vi "NIIE_PictureControl_MouseUp.vi"(7 "Finalize Movement":bool, 8 "Error":errorcluster, 10 "Coords":T5, 11 "Data":T1={"Class"={"Ants"=refnum, "Layer"=refnum, "Templates"=refnum, "Icon"=refnum, "Glyph"=refnum, "Settings"=refnum, "Tools"=refnum}, "Ref"={"Add Layer"=refnum, "Remove Layer"=refnum, "Line Text"=[], "Body Text Spec"=refnum, "DNL_Font"=refnum, "glyph path str"=refnum, "templates path str"=refnum, "Arrow Up"=refnum, "Arrow Down"=refnum, "IE VI Ref"=refnum, "Glyphs tree"=refnum, "Templates tree"=refnum, "Layer Icon Text"=refnum, "Layer Template"=refnum, "Clipboard"=refnum, "BW icon in"=refnum, "Color icon in"=refnum, "Layer Clust"=refnum, "Body Text"=refnum, "DNL_Framework Templates"=refnum, "Search Templates"=refnum, "TextMarker"=refnum, "Tab Control"=refnum, "Search Glyphs"=refnum, "Line Color"=refnum, "DNL_Glyphs []"=refnum, "Fill Color"=refnum, "Tools"=refnum, "Glyphs tree"=refnum, "Icon"=refnum, "Preview"=refnum, "Ants"=refnum, "Terminals"=refnum, "menu reference"=refnum, "LayerNames"=[], "GlyphLoadAnimation"=refnum, "TemplateLoadAnimation"=refnum, "refreshGlyphs"=refnum, "refreshTemplates"=refnum}, "Support"={"AntsRect"={"left"=0, "top"=0, "right"=0, "bottom"=0}, "Mouse Move Coords"={"Horizontal"=0, "Vertical"=0}, "Mouse Down Coords"={"Horizontal"=0, "Vertical"=0}, "Temp Coord"={"Horizontal"=0, "Vertical"=0}, "Action"=enum."Default", "Edge Color"=4914962, "Fill Color"=16860, "Mouse Down?"=FALSE, "Draft Mode?"=FALSE, "Temp Icon"=bytes[3102], "CTRL Pressed"=FALSE, "Move Selection?"=FALSE, "AntsRect Orig"={"left"=0, "top"=0, "right"=0, "bottom"=0}, "Text"="", "TM Set?"=FALSE, "Mouse inside icon?"=FALSE, "Tool (old value)"=0, "Pencil Move Color"=0, "Swap Colors?"=FALSE, "Shift pressed?"=FALSE}}) -> (0 "Error Out":errorcluster, 3 "Data Out":T1={"Class"={"Ants"=refnum, "Layer"=refnum, "Templates"=refnum, "Icon"=refnum, "Glyph"=refnum, "Settings"=refnum, "Tools"=refnum}, "Ref"={"Add Layer"=refnum, "Remove Layer"=refnum, "Line Text"=[], "Body Text Spec"=refnum, "DNL_Font"=refnum, "glyph path str"=refnum, "templates path str"=refnum, "Arrow Up"=refnum, "Arrow Down"=refnum, "IE VI Ref"=refnum, "Glyphs tree"=refnum, "Templates tree"=refnum, "Layer Icon Text"=refnum, "Layer Template"=refnum, "Clipboard"=refnum, "BW icon in"=refnum, "Color icon in"=refnum, "Layer Clust"=refnum, "Body Text"=refnum, "DNL_Framework Templates"=refnum, "Search Templates"=refnum, "TextMarker"=refnum, "Tab Control"=refnum, "Search Glyphs"=refnum, "Line Color"=refnum, "DNL_Glyphs []"=refnum, "Fill Color"=refnum, "Tools"=refnum, "Glyphs tree"=refnum, "Icon"=refnum, "Preview"=refnum, "Ants"=refnum, "Terminals"=refnum, "menu reference"=refnum, "LayerNames"=[], "GlyphLoadAnimation"=refnum, "TemplateLoadAnimation"=refnum, "refreshGlyphs"=refnum, "refreshTemplates"=refnum}, "Support"={"AntsRect"={"left"=0, "top"=0, "right"=0, "bottom"=0}, "Mouse Move Coords"={"Horizontal"=0, "Vertical"=0}, "Mouse Down Coords"={"Horizontal"=0, "Vertical"=0}, "Temp Coord"={"Horizontal"=0, "Vertical"=0}, "Action"=enum."Default", "Edge Color"=4914962, "Fill Color"=16860, "Mouse Down?"=FALSE, "Draft Mode?"=FALSE, "Temp Icon"=bytes[3102], "CTRL Pressed"=FALSE, "Move Selection?"=FALSE, "AntsRect Orig"={"left"=0, "top"=0, "right"=0, "bottom"=0}, "Text"="", "TM Set?"=FALSE, "Mouse inside icon?"=FALSE, "Tool (old value)"=0, "Pencil Move Color"=0, "Swap Colors?"=FALSE, "Shift pressed?"=FALSE}})   [LabVIEW 2021]
uses:
  <vilib>/Utility/miscctls.llb/LVPoint32TypeDef.ctl
  Controls/IE Data.ctl
  Class/Ants/Ants.lvclass
  Class/FakedArray/FakedArray.lvclass
  Class/Icon Library/Glyph.lvclass
  Class/Settings/Settings.lvclass
  Class/Tools/Tools Paint.lvclass
  vi.lib/LabVIEW Icon API/lv_icon/Classes/Icon/Icon.lvclass
  Controls/IE Classes.ctl
  Controls/References Cluster.ctl
  Controls/SupportClass.ctl
  Controls/ENUM_SupportClass_Action.ctl
  vi.lib/LabVIEW Icon API/lv_icon/Controls/IEColor.ctl
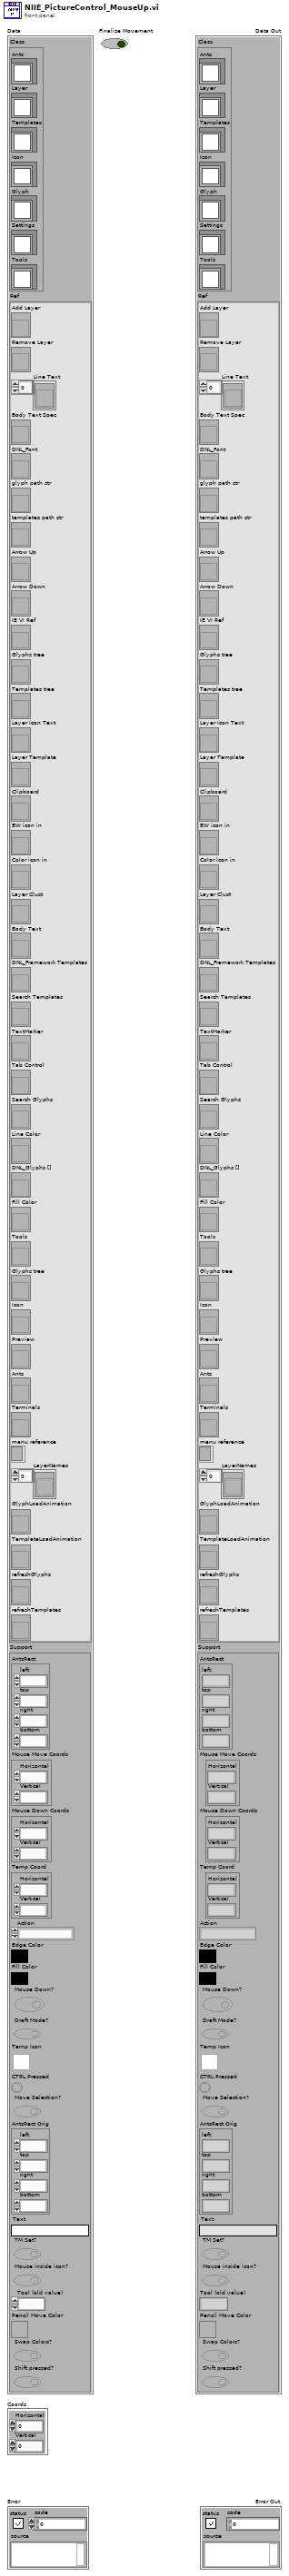
[diagram p1: front panel]
types:
  T1 = typedef "IE Data.ctl" = cluster{"Class":T2, "Ref":T3, "Support":T4}
  T2 = typedef "IE Classes.ctl" = cluster{"Ants":refnum<class "Ants.lvclass">, "Layer":refnum<class "FakedArray.lvclass">, "Templates":refnum<class "FakedArray.lvclass">, "Icon":refnum<class "Icon.lvclass">, "Glyph":refnum<class "Glyph.lvclass">, "Settings":refnum<class "Settings.lvclass">, "Tools":refnum<class "Tools Paint.lvclass">}
  T3 = typedef "References Cluster.ctl" = cluster{"Add Layer":refnum<vi>, "Remove Layer":refnum<vi>, "Line Text":refnum<vi>[], "Body Text Spec":refnum<vi>, "DNL_Font":refnum<vi>, "glyph path str":refnum<vi>, "templates path str":refnum<vi>, "Arrow Up":refnum<vi>, "Arrow Down":refnum<vi>, "IE VI Ref":refnum<vi>, "Glyphs tree":refnum<vi>, "Templates tree":refnum<vi>, "Layer Icon Text":refnum<vi>, "Layer Template":refnum<vi>, "Clipboard":refnum<vi>, "BW icon in":refnum<vi>, "Color icon in":refnum<vi>, "Layer Clust":refnum<vi>, "Body Text":refnum<vi>, "DNL_Framework Templates":refnum<vi>, "Search Templates":refnum<vi>, "TextMarker":refnum<vi>, "Tab Control":refnum<vi>, "Search Glyphs":refnum<vi>, "Line Color":refnum<vi>, "DNL_Glyphs []":refnum<vi>, "Fill Color":refnum<vi>, "Tools":refnum<vi>, "Glyphs tree":refnum<vi>, "Icon":refnum<vi>, "Preview":refnum<vi>, "Ants":refnum<vi>, "Terminals":refnum<vi>, "menu reference":refnum<k9>, "LayerNames":refnum<vi>[], "GlyphLoadAnimation":refnum<vi>, "TemplateLoadAnimation":refnum<vi>, "refreshGlyphs":refnum<vi>, "refreshTemplates":refnum<vi>}
  T4 = typedef "SupportClass.ctl" = cluster{"AntsRect":cluster{"left":i16, "top":i16, "right":i16, "bottom":i16}, "Mouse Move Coords":T5, "Mouse Down Coords":T5, "Temp Coord":T5, "Action":T6, "Edge Color":T7, "Fill Color":T7, "Mouse Down?":bool, "Draft Mode?":bool, "Temp Icon":picture, "CTRL Pressed":bool, "Move Selection?":bool, "AntsRect Orig":cluster{"left":i16, "top":i16, "right":i16, "bottom":i16}, "Text":string, "TM Set?":bool, "Mouse inside icon?":bool, "Tool (old value)":u32, "Pencil Move Color":u32, "Swap Colors?":bool, "Shift pressed?":bool}
  T5 = typedef "LVPoint32TypeDef.ctl" = cluster{"Horizontal":i32, "Vertical":i32}
  T6 = typedef "ENUM_SupportClass_Action.ctl" = enum16{"Default", "Move Selection", "Glyph Library", "Tool"}
  T7 = typedef "IEColor.ctl" = u32
  T8 = cluster{"left":i16, "top":i16, "right":i16, "bottom":i16}
  T9 = cluster{"Horizontal":i32, "Vertical":i32, "Vertical 2":i32, "Vertical 3":i32}
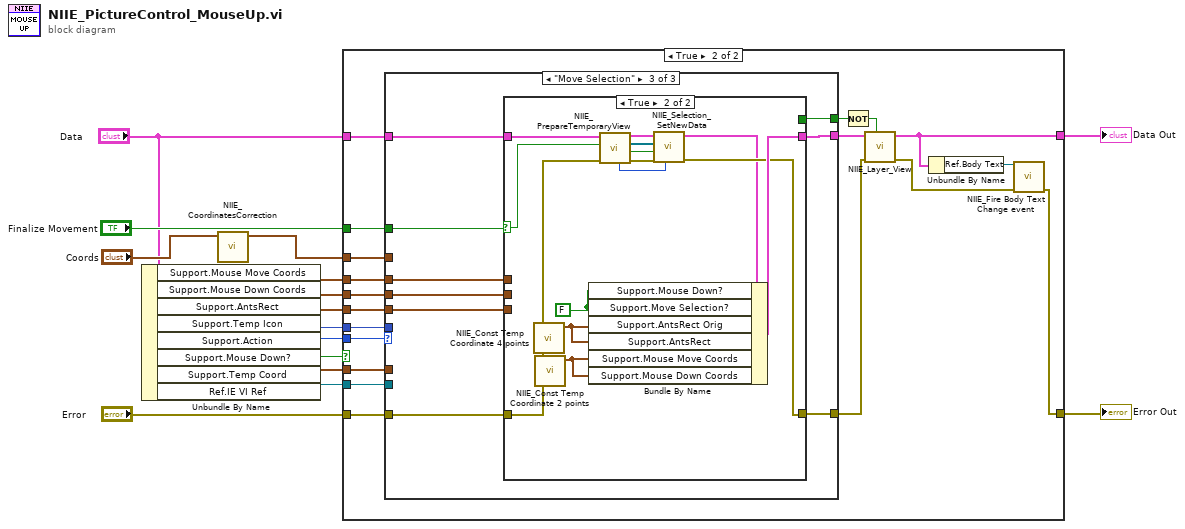
[diagram p0: block diagram]
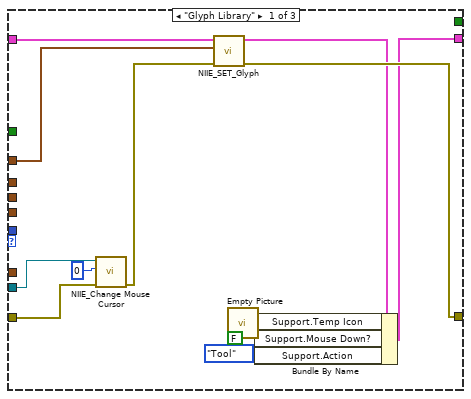
[diagram p3: hidden frame]
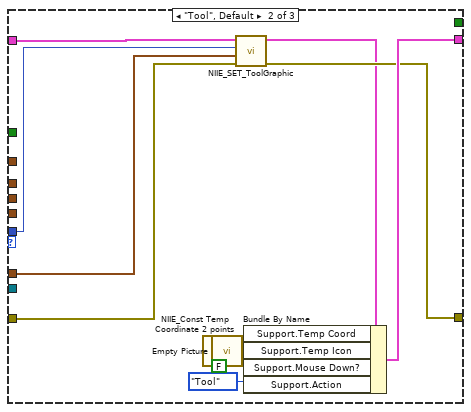
[diagram p4: hidden frame]
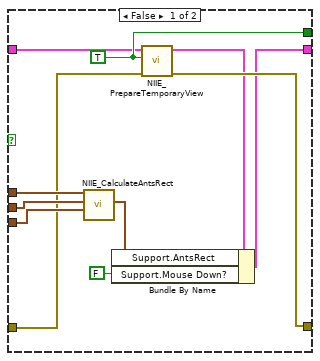
[diagram p5: hidden frame]
diagram:
  n1 = Unbundle By Name("Data") -> ("Support.Mouse Move Coords"=w6:T5, "Support.Mouse Down Coords"=w7:T5, "Support.AntsRect"=w8:T8, "Support.Temp Icon"=w13:picture, "Support.Action"=w11:T6, "Support.Mouse Down?"=w12:bool, "Support.Temp Coord"=w15:T5, "Ref.IE VI Ref"=w1:refnum<vi>)
  n2 = call "NIIE_CoordinatesCorrection.vi"("Coordinates In"="Coords") -> ("Corrected Out"=w14:T5)  [unwired: 10 out]
  n3 = case shown="True" w12 {
    tunnel: w11 -> [_ w36]
    tunnel: "Error" -> [w17 w35]
    tunnel: w13 -> [_ w34]
    tunnel: w14 -> [_ w33]
    tunnel: [w17 w20] -> w3
    tunnel: w15 -> [_ w32]
    tunnel: "Finalize Movement" -> [_ w30]
    tunnel: w8 -> [_ w29]
    tunnel: w7 -> [_ w28]
    tunnel: w6 -> [_ w27]
    tunnel: "Data" -> [w16 w24]
    tunnel: [w16 w19] -> w2
    tunnel: w1 -> [_ w22]
    frame False {
    }
    frame True {
      n4 = case shown="\"Move Selection\"" w36 {
        tunnel: w35 -> [w43 w51 w68]
        tunnel: w34 -> [_ w55 _]
        tunnel: w33 -> [w48 _ _]
        tunnel: [w37 w57 w66] -> w23
        tunnel: [w44 w54 w67] -> w31
        tunnel: w32 -> [_ w53 _]
        tunnel: w30 -> [_ _ w65]
        tunnel: w29 -> [_ _ w62]
        tunnel: w28 -> [_ _ w63]
        tunnel: w27 -> [_ _ w64]
        tunnel: [_ _ w61] -> w25
        tunnel: w24 -> [w41 w50 w60]
        tunnel: w22 -> [w39 _ _]
        frame "Glyph Library" {
          n5 = call "NIIE_Change Mouse Cursor.vi"("error in (no error)"=w43, "icon"=u16 0, "VI reference (current VI)"=w39) -> ("error out"=w42:errorcluster)  [unwired: 8 out]
          n6 = call "NIIE_SET_Glyph.vi"("Error"=w42, "Coordinates"=w48, "Data"=w41) -> ("Error Out"=w44:errorcluster, "Data Out"=w38:T1)  [unwired: 7 out]
          n7 = call "Empty Picture"() -> ("empty picture"=w45:picture)
          n8 = Bundle By Name(cluster=w38, "Support.Temp Icon"=w45, "Support.Mouse Down?"=FALSE ("Mouse Down?"), "Support.Action"=ENUM_SupportClass_Action."Tool" ("Action")) -> (w37:T1)
        }
        frame "Tool", Default {
          n9 = call "NIIE_Const Temp Coordinate 2 points.vi"() -> ("Const Temp Coordinate"=w52:T5)  [unwired: 11 out]
          n10 = call "Empty Picture"() -> ("empty picture"=w56:picture)
          n11 = call "NIIE_SET_ToolGraphic.vi"("Error"=w51, "Temp Coord"=w53, "Temp Icon"=w55, "Data"=w50) -> ("Error Out"=w54:errorcluster, "Data Out"=w49:T1)  [unwired: 6 out]
          n12 = Bundle By Name(cluster=w49, "Support.Temp Coord"=w52, "Support.Temp Icon"=w56, "Support.Mouse Down?"=FALSE ("Mouse Down?"), "Support.Action"=ENUM_SupportClass_Action."Tool" ("Action")) -> (w57:T1)
        }
        frame "Move Selection" {
          n13 = case shown="True" w65 {
            selector: w65 -> [_ w90]
            tunnel: w68 -> [w74 w86]
            tunnel: [w73 w85] -> w67
            tunnel: [w69 w89] -> w66
            tunnel: w64 -> [w78 _]
            tunnel: w63 -> [w77 _]
            tunnel: w62 -> [w76 _]
            tunnel: [w72 _] -> w61
            tunnel: w60 -> [w71 w82]
            frame False {
              w72 = TRUE ("Valid Selection?")
              n14 = call "NIIE_CalculateAntsRect.vi"("AntsRect"=w76, "Mouse Down Coords"=w77, "Mouse Move Coords"=w78) -> ("Rect"=w75:cluster{i32, i32, i32, i32})  [unwired: 8 out]
              n15 = call "NIIE_PrepareTemporaryView.vi"("Error"=w74, "Valid Selection?"=w72, "Data"=w71) -> ("Error Out"=w73:errorcluster, "Data Out"=w70:T1)  [unwired: 2 in, 5 out]
              n16 = Bundle By Name(cluster=w70, "Support.AntsRect"=w75, "Support.Mouse Down?"=FALSE ("Mouse Down?")) -> (w69:T1)
            }
            frame True {
              w88 = FALSE ("Move Selection?")
              n17 = call "NIIE_Const Temp Coordinate 4 points.vi"() -> ("Const Temp Coordinate"=w84:T9)  [unwired: 11 out]
              n18 = call "NIIE_Const Temp Coordinate 2 points.vi"() -> ("Const Temp Coordinate"=w83:T5)  [unwired: 11 out]
              n19 = call "NIIE_PrepareTemporaryView.vi"("Error"=w86, "Valid Selection?"=w90, "Data"=w82) -> ("Error Out"=w87:errorcluster, "Highlighted? Out"=w92:bool, "All Layers Out"=w93:refnum<class "Layer.lvclass">[], "Data Out"=w81:T1, "#Active Layer Out"=w91:i32)  [unwired: 2 in, 2 out]
              n20 = call "NIIE_Selection_SetNewData.vi"("#Active Layer"=w91, "Error"=w87, "Highlighted?"=w92, "All Layers"=w93, "Data"=w81) -> ("Error Out"=w85:errorcluster, "Data Out"=w80:T1)  [unwired: 1 in, 3 out]
              n21 = Bundle By Name(cluster=w80, "Support.Mouse Down?"=w88, "Support.Move Selection?"=w88, "Support.AntsRect Orig"=w84, "Support.AntsRect"=w84, "Support.Mouse Move Coords"=w83, "Support.Mouse Down Coords"=w83) -> (w89:T1)
            }
          }
        }
      }
      n22 = Not(x=w25) -> (.not. x?=w26:bool)
      n23 = call "NIIE_Layer_View.vi"("Add To Undo?"=w26, "Error"=w31, "Data"=w23) -> ("Error Out"=w21:errorcluster, "Data Out"=w19:T1)  [unwired: 2 in, 5 out]
      n24 = Unbundle By Name(w19) -> ("Ref.Body Text"=w18:refnum<vi>)
      n25 = call "NIIE_Fire Body Text Change event.vi"("error in"=w21, "Ref.Body Text"=w18) -> ("error out"=w20:errorcluster)  [unwired: 9 in]
    }
  }
  "Error Out" <- w3
  "Data Out" <- w2
